vi "CastDependenciesClusterToArray.vi"(11 "Dependencies Cluster":variant) -> (1 "Shared Resources":bool[](array[boolean]), 2 "Dependencies Names":string[](array[string]), 3 "Dependencies Array":refnum<class "SMO.lvclass">[](array[class]))   [LabVIEW 2021, in "smo.lvlib" / "SMO.lvclass"]
uses:
  SMO.lvclass
  SMO.lvclass/SMO.ctl
  <vilib>/Utility/VariantDataType/VariantType.lvlib
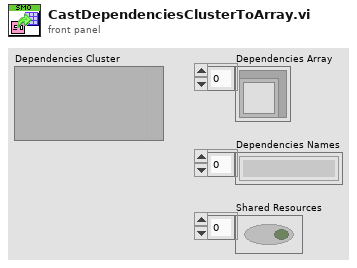
[diagram p1: front panel]
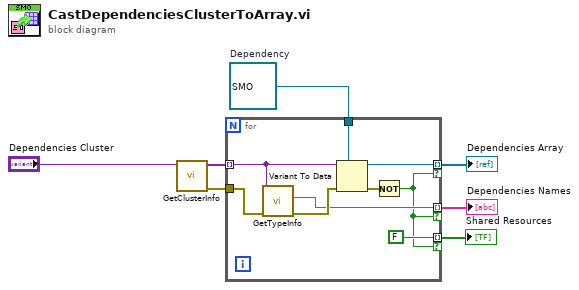
[diagram p0: block diagram]
diagram:
  w2 = refnum<class "SMO.lvclass"> refnum  # Dependency
  n1 = call <vilib>:"GetClusterInfo.vi"("Variant"="Dependencies Cluster") -> ("error out"=w4:errorcluster, "Cluster Elements"=w1:variant[])  [unwired: 9 in]
  n2 = for {
    tunnel: w1 -> [w11] mode=indexing
    tunnel: w2 -> [w16]
    tunnel: [w15] -> w3 mode=indexing if=w8
    tunnel: w4 -> [w13]
    tunnel: [w10] -> w5 mode=indexing if=w8
    tunnel: [FALSE] -> w7 mode=indexing if=w8
    n3 = call <vilib>:"GetTypeInfo.vi"("error in (no error)"=w13, "Variant"=w11) -> ("error out"=w12:errorcluster, "Name"=w10:string)  [unwired: 5 in, 3 out]
    n4 = Variant To Data(error in=w12, type=w16, Variant=w11) -> (data=w15:refnum<class "SMO.lvclass">, error out=w14:errorcluster)
    n5 = Not(x=w14) -> (.not. x?=w8:bool)
  }
  "Shared Resources" <- w7
  "Dependencies Names" <- w5
  "Dependencies Array" <- w3
